vi "Gif.Main.vi"(0 "file path":path, 9 "bgcolor":u32(colorbox)=16777226, 11 "error in (no error)":errorcluster, 12 "image index":i32) -> (4 "fileData":string, 6 "time":u32[](array[numeric]), 8 "images out":picture[](array[picture]), 13 "image data":T1, 14 "image size":cluster{"Width":u32, "Height":u32}, 15 "error out":errorcluster)   [LabVIEW 2019]
doc: "This VI reads all images from a gif file.\nCurrently it can only read from version 89a.\nInterlaced images are not taken into account.\n\nThe outputs are an array of all delay times, an array of all images, the image size and an error cluster.\n\nVersion 01.01\nMike Schröder"
uses:
  <vilib>/picture/picture.llb/imagedata.ctl
panel:
  out "color table":u32[](array[colorbox])
  out "Version":string
  out "Signature":string
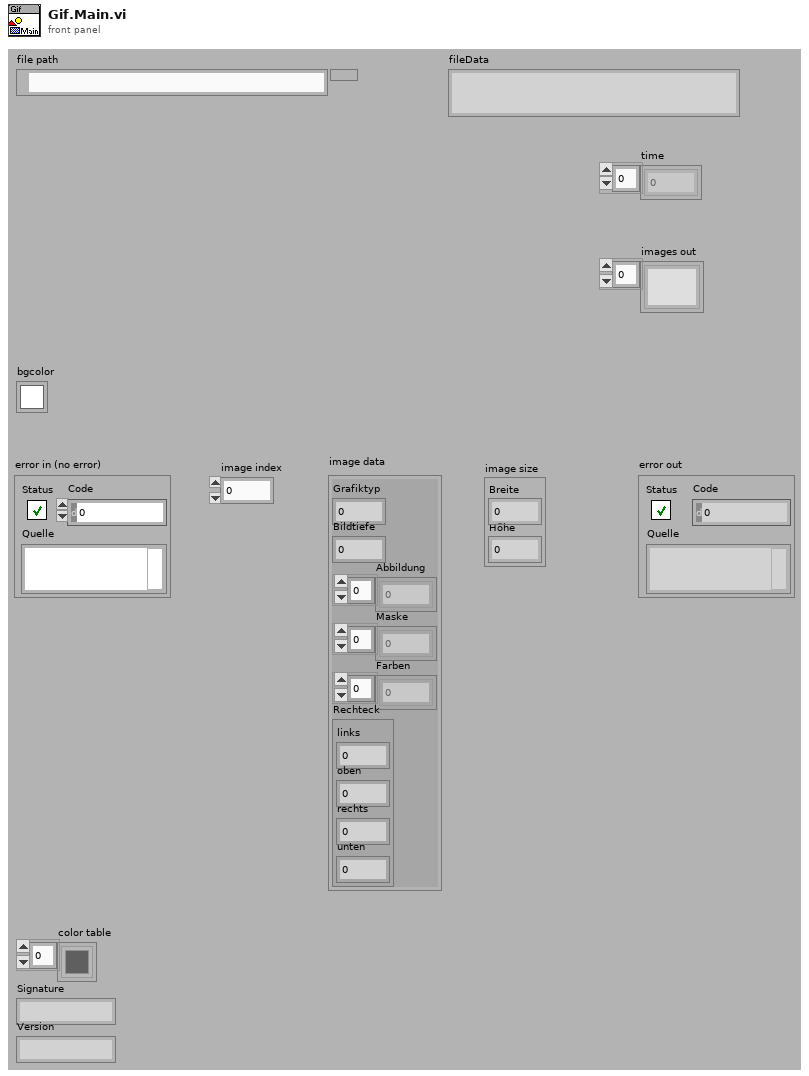
[diagram p1: front panel]
types:
  T1 = typedef "imagedata.ctl" = cluster{"image type":i32, "image depth":i32, "image":u8[], "mask":u8[], "colors":u32[], "Rectangle":cluster{"left":i16, "top":i16, "right":i16, "bottom":i16}}
  T2 = enum16{"deny read/write", "deny write-only", "deny none"}
  T3 = enum16{"read/write", "read-only", "write-only", "write-only (truncate)"}
  T4 = typedef "Gif.LogicalScreenDescriptior.ctl" = cluster{"Logical Screen Width":u16, "Logical Screen Height":u16, "Global Color Table Flag":u8, "Color Resolution":u8, "Sort Flag":u8, "Size of Global Color Table":u8, "Background Color Index":u8, "Pixel Aspect Ratio":u8}
  T5 = typedef "Gif.GraphicControlExtension.ctl" = cluster{"Reserved":u8, "Disposal Method":u8, "User Input Flag":u8, "Transparent Color Flag":u8, "Delay Time":u16, "Transparent Color Index":u8}
  T6 = typedef "Gif.ImageDescriptor.ctl" = cluster{"Image Left Position":u16, "Image Top Position":u16, "Image Width":u16, "Image Height":u16, "Local Color Table Flag":u8, "Interlace Flag":u8, "Sort Flag":u8, "Reserved":u8, "Size Of Local Color Table":u8}
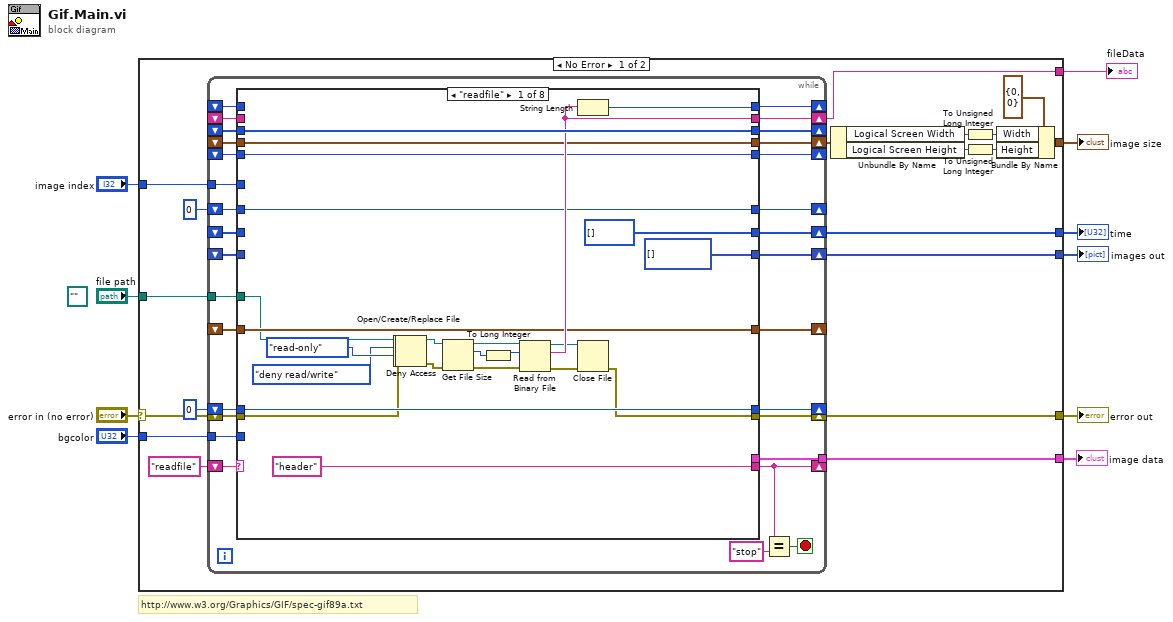
[diagram p0: block diagram]
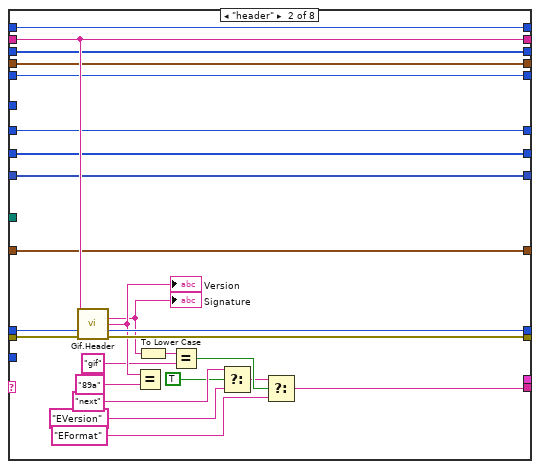
[diagram p2: hidden frame]
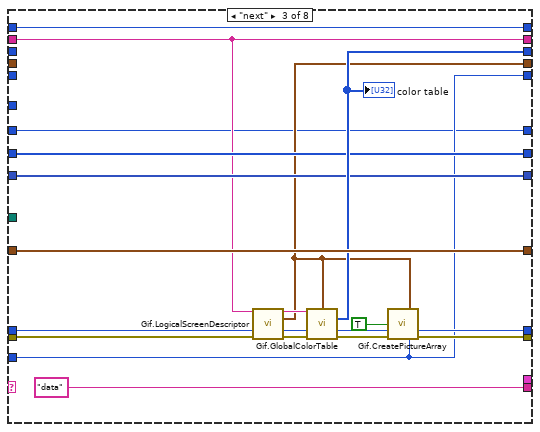
[diagram p3: hidden frame]
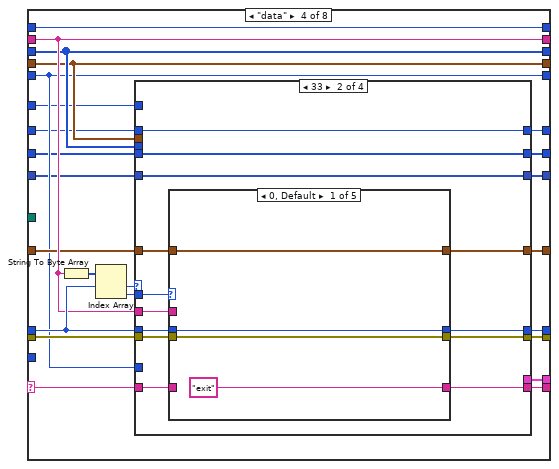
[diagram p4: hidden frame]
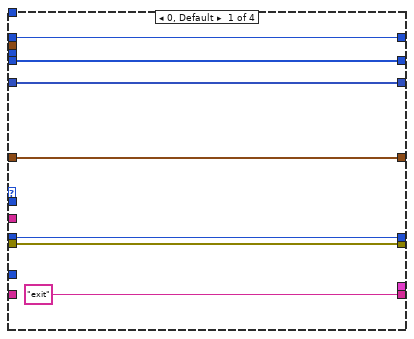
[diagram p5: hidden frame]
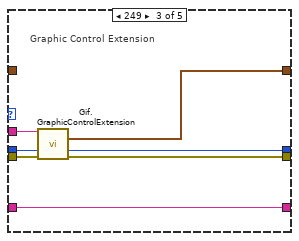
[diagram p7: hidden frame]
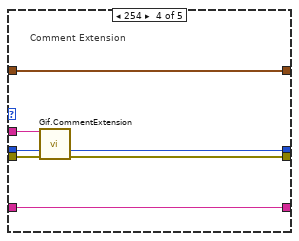
[diagram p8: hidden frame]
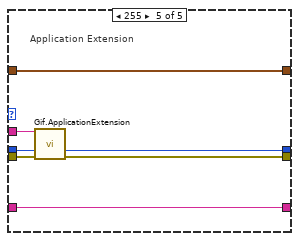
[diagram p9: hidden frame]
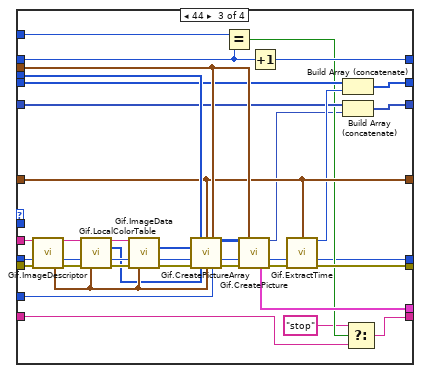
[diagram p10: hidden frame]
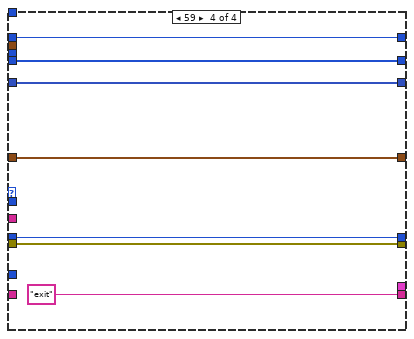
[diagram p11: hidden frame]
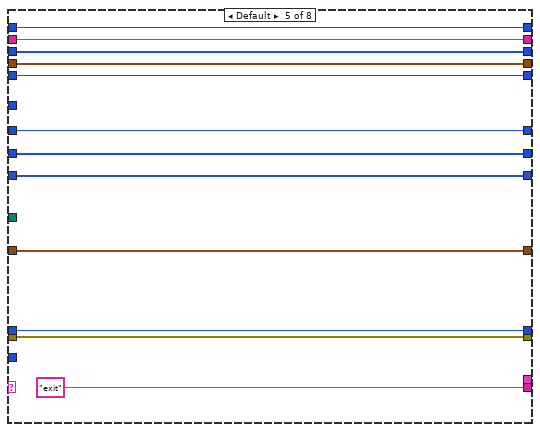
[diagram p12: hidden frame]
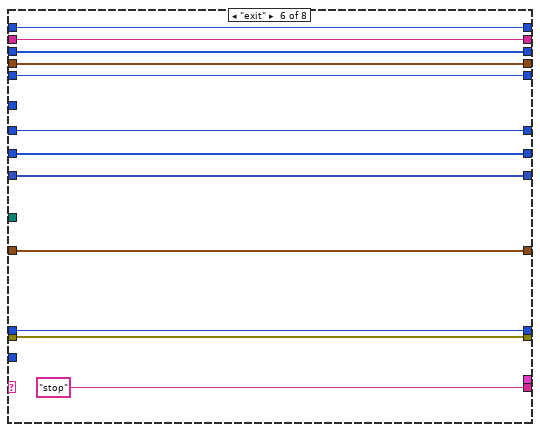
[diagram p13: hidden frame]
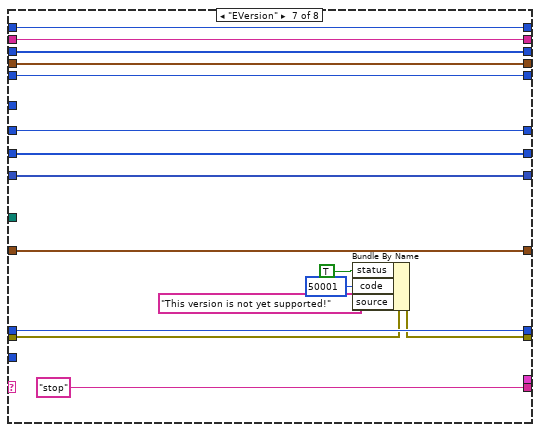
[diagram p14: hidden frame]
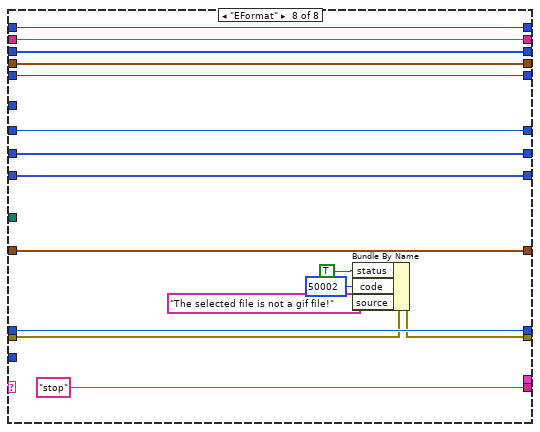
[diagram p15: hidden frame]
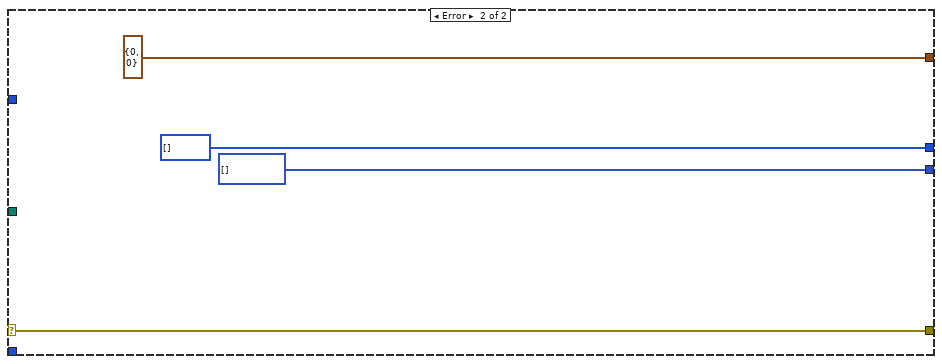
[diagram p16: hidden frame]
diagram:
  (unwired) path "" ("file path")
  # "http://www.w3.org/Graphics/GIF/spec-gif89a.txt"
  n1 = case shown="No Error" "error in (no error)" {
    selector: "error in (no error)" -> [w15 w309]
    tunnel: [w27 u32[] []] -> w10
    tunnel: [w26 picture[] []] -> w2
    tunnel: "bgcolor" -> [w24 _]
    tunnel: "file path" -> [w23 _]
    tunnel: [w22 w309] -> w7
    tunnel: [w16 cluster{"Width":u32, "Height":u32} {"Width"=0, "Height"=0} ("Größe des Darstellungsbereichs")] -> w6
    tunnel: "image index" -> [w13 _]
    tunnel: [w12 _] -> w3
    tunnel: [w11 _] -> w1
    frame No Error {
      n2 = while {
        shift-right: [w50] -> _
        shift-left: "readfile" -> [w59]
        shift-right: [w58] -> _
        shift-left: _ -> [w56]
        shift-right: [w57] -> w11
        shift-left: _ -> [w55]
        shift-right: [w53] -> w22
        shift-left: w15 -> [w54]
        shift-right: [w51] -> _
        shift-left: 0 ("offset (0)") -> [w52]
        shift-right: [w47] -> _
        shift-left: _ -> [w46]
        shift-right: [w45] -> _
        shift-left: _ -> [w44]
        shift-right: [w43] -> w25
        shift-left: _ -> [w42]
        shift-right: [w41] -> _
        shift-left: _ -> [w40]
        shift-right: [w38] -> w27
        shift-left: _ -> [w39]
        shift-right: [w36] -> w26
        shift-left: _ -> [w37]
        tunnel: w24 -> [w35]
        tunnel: w23 -> [w34]
        shift-right: [w31] -> _
        shift-left: 0 ("offset (0)") -> [w32]
        tunnel: w13 -> [w30]
        tunnel: [w33] -> w12
        stop <- w48 stop-if-true
        n3 = case shown="\"readfile\"" w59 {
          selector: w59 -> [_ _ _ w145 _ _ _ _]
          tunnel: [w85 w110 w130 w154 w261 w273 w289 w305] -> w58
          tunnel: [w81 w108 w114 w144 w260 w272 w288 w304] -> w57
          tunnel: w56 -> [_ w110 w130 w154 w261 w273 w289 w305]
          tunnel: w55 -> [_ w108 w114 w144 w260 w272 w288 w304]
          tunnel: ["header" w89 "data" w146 "exit" "stop" "stop" "stop"] -> w50
          tunnel: w54 -> [w73 w109 w113 w149 w258 w270 w279 w295]
          tunnel: [w60 w103 w117 w148 w258 w270 w278 w294] -> w53
          tunnel: w52 -> [w83 w107 w112 w150 w257 w269 w286 w302]
          tunnel: [w83 w102 w119 w147 w257 w269 w286 w302] -> w51
          tunnel: [w82 w101 w124 w143 w256 w268 w285 w301] -> w47
          tunnel: w46 -> [w82 w101 _ w143 w256 w268 w285 w301]
          tunnel: [w78 w106 w128 w142 w255 w267 w284 w300] -> w45
          tunnel: w44 -> [w78 w106 w128 w141 w255 w267 w284 w300]
          tunnel: [w77 w100 w116 w140 w254 w266 w283 w299] -> w43
          tunnel: w42 -> [w77 w100 _ w140 w254 w266 w283 w299]
          tunnel: [w76 w99 w115 w139 w253 w265 w282 w298] -> w41
          tunnel: w40 -> [w76 w99 _ w139 w253 w265 w282 w298]
          tunnel: w39 -> [_ w105 w123 w138 w252 w264 w281 w297]
          tunnel: [u32[] [] w105 w123 w137 w252 w264 w281 w297] -> w38
          tunnel: w37 -> [_ w104 w122 w136 w251 w263 w280 w296]
          tunnel: [picture[] [] w104 w122 w135 w251 w263 w280 w296] -> w36
          tunnel: w35 -> [_ _ w115 _ _ _ _ _]
          tunnel: w34 -> [w74 _ _ _ _ _ _ _]
          tunnel: [_ _ _ w134 _ _ _ _] -> w33
          tunnel: w32 -> [w72 w86 w111 w133 w250 w262 w274 w290]
          tunnel: [w72 w86 w111 w132 w250 w262 w274 w290] -> w31
          tunnel: w30 -> [_ _ _ w131 _ _ _ _]
          frame "readfile" {
            n4 = Open/Create/Replace File(file path (use dialog)=w74, error in=w73, access (0:read/write)=T3."read-only" ("open mode (0)")) -> (refnum out=w63:refnum<file>, error out=w64:errorcluster)  [unwired: 3 in, 1 out]
            n5 = Deny Access(4:w64, 6:T2."deny read/write" ("deny mode (2)"), 7:w63) -> (0:w69:errorcluster, 3:w70:refnum<file>)
            n6 = Get File Size(file=w70, error in=w69) -> (refnum out=w79:refnum<file>, size (in bytes)=w65:i64, 0:w80:errorcluster)
            n7 = To Long Integer(number=w65) -> (32bit integer=w68:i32)
            n8 = Read from Binary File(8:w80, 10:w68, 11:w79) -> (0:w61:errorcluster, 2:w81:string, 3:w62:refnum<file>)  [unwired: 3 in, 1 out]
            n9 = String Length(string=w81) -> (length=w85:i32)
            n10 = Close File(refnum=w62, error in=w61) -> (error out=w60:errorcluster)  [unwired: 1 out]
          }
          frame "header" {
            n11 = call "Gif.Header.vi"("data"=w108, "offset"=w107, "error in (no error)"=w109) -> ("Signature"=w94:string, "Version"=w98:string, "offset out"=w102:i32, "error out"=w103:errorcluster)  [unwired: 1 in, 8 out]
            "Signature" <- w94
            "Version" <- w98
            n12 = Equal?(x=w98, y="89a") -> ()  [unwired: 1 out]
            n13 = To Lower Case(string=w94) -> (all lower case string=w93:string)
            n14 = Equal?(x=w93, y="gif") -> (x = y?=w91:bool)
            n15 = Select(t="next", s=TRUE, f="EVersion") -> (s? t:f=w90:string)
            n16 = Select(t=w90, s=w91, f="EFormat") -> (s? t:f=w89:string)
          }
          frame "next" {
            n17 = call "Gif.LogicalScreenDescriptor.vi"("data"=w114, "offset"=w112, "error in (no error)"=w113) -> ("data out"=w125:string, "Logical Screen Descriptor"=w116:T4, "offset out"=w126:i32, "error out"=w127:errorcluster)  [unwired: 9 out]
            n18 = call "Gif.GlobalColorTable.vi"("data"=w125, "Logical Screen Descriptor"=w116, "offset"=w126, "error in (no error)"=w127) -> ("global color table"=w124:u32[], "offset out"=w120:i32, "error out"=w118:errorcluster)  [unwired: 1 in, 8 out]
            "color table" <- w124
            n19 = call "Gif.CreatePictureArray.vi"("Logical Screen Description"=w116, "init"=TRUE, "offset"=w120, "error in (no error)"=w118, "bgcolor"=w115) -> ("offset out"=w119:i32, "error out"=w117:errorcluster)  [unwired: 5 in, 4 out]
          }
          frame "data" {
            n20 = String To Byte Array(string=w144) -> (unsigned byte array=w153:u8[])
            n21 = Index Array(array=w153, index #1=w150) -> (element #1=w152:u8, element #2=w151:u8)  [unwired: 1 in]
            n22 = case shown="33" w152 {
              tunnel: w151 -> [_ w174 _ _]
              tunnel: w150 -> [w160 w170 w241 w248]
              tunnel: w149 -> [w161 w169 w242 w247]
              tunnel: [w161 w168 w216 w247] -> w148
              tunnel: [w160 w171 w206 w248] -> w147
              tunnel: ["exit" w173 w208 "exit"] -> w146
              tunnel: w145 -> [_ w172 w210 _]
              tunnel: w144 -> [_ w167 w240 _]
              tunnel: w143 -> [_ _ w226 _]
              tunnel: [w158 w166 w224 w246] -> w142
              tunnel: w141 -> [w158 w165 w224 w246]
              tunnel: w140 -> [_ _ w225 _]
              tunnel: w139 -> [_ _ w223 _]
              tunnel: w138 -> [w157 w164 w222 w245]
              tunnel: [w157 w164 w220 w245] -> w137
              tunnel: w136 -> [w156 w163 w219 w244]
              tunnel: [w156 w163 w218 w244] -> w135
              tunnel: [_ _ w214 _] -> w134
              tunnel: w133 -> [w155 w162 w204 w243]
              tunnel: [w155 w162 w212 w243] -> w132
              tunnel: w131 -> [_ _ w213 _]
              frame 0, Default {
              }
              frame 33 {
                n23 = case shown="0, Default" w174 {
                  tunnel: ["exit" w182 w189 w196 w203] -> w173
                  tunnel: w172 -> [_ w182 w189 w196 w203]
                  tunnel: [w177 w181 w185 w193 w201] -> w171
                  tunnel: w170 -> [w177 w181 w187 w194 w202]
                  tunnel: w169 -> [w176 w180 w188 w195 w200]
                  tunnel: [w176 w180 w186 w192 w199] -> w168
                  tunnel: w167 -> [_ _ w184 w191 w198]
                  tunnel: [w175 w179 w183 w190 w197] -> w166
                  tunnel: w165 -> [w175 w179 _ w190 w197]
                  frame 0, Default {
                  }
                  frame 1 {
                  }
                  frame 249 {
                    # "Graphic Control Extension"
                    n24 = call "Gif.GraphicControlExtension.vi"("data"=w184, "offset"=w187, "error in (no error)"=w188) -> ("GraphicControlExtension"=w183:T5, "offset out"=w185:i32, "error out"=w186:errorcluster)  [unwired: 10 out]
                  }
                  frame 254 {
                    # "Comment Extension"
                    n25 = call "Gif.CommentExtension.vi"("data"=w191, "offset"=w194, "error in (no error)"=w195) -> ("offset out"=w193:i32, "error out"=w192:errorcluster)  [unwired: 11 out]
                  }
                  frame 255 {
                    # "Application Extension"
                    n26 = call "Gif.ApplicationExtension.vi"("data"=w198, "offset"=w202, "error in (no error)"=w200) -> ("offset out"=w201:i32, "error out"=w199:errorcluster)  [unwired: 11 out]
                  }
                }
              }
              frame 44 {
                n27 = call "Gif.ImageDescriptor.vi"("data"=w240, "offset"=w241, "error in (no error)"=w242) -> ("data out"=w237:string, "offset out"=w238:i32, "ImageDescriptor"=w228:T6, "error out"=w239:errorcluster)  [unwired: 9 out]
                n28 = call "Gif.LocalColorTable.vi"("data"=w237, "offset"=w238, "error in (no error)"=w239, "ImageDescriptor"=w228) -> ("data out"=w234:string, "local color table"=w227:u32[], "offset out"=w235:i32, "error out"=w236:errorcluster)  [unwired: 5 in, 3 out]
                n29 = call "Gif.ImageData.vi"("data"=w234, "offset"=w235, "error in (no error)"=w236, "ImageDescriptor"=w228) -> ("Index Array"=w232:i32[], "offset out"=w207:i32, "error out"=w233:errorcluster)  [unwired: 1 in, 8 out]
                n30 = call "Gif.CreatePictureArray.vi"("gloal color table"=w226, "GraphicControlExtension"=w224, "Logical Screen Description"=w225, "Index Array"=w232, "offset"=w207, "error in (no error)"=w233, "local color table"=w227, "ImageDescriptor"=w228, "bgcolor"=w223) -> ("image out"=w229:u32[][], "offset out"=w230:i32, "error out"=w231:errorcluster)  [unwired: 1 in, 3 out]
                n31 = Equal?(x=w213, y=w204) -> (x = y?=w211:bool)
                n32 = call "Gif.CreatePicture.vi"("image in"=w229, "Logical Screen Description"=w225, "offset"=w230, "error in (no error)"=w231) -> ("image out"=w205:picture, "offset out"=w215:i32, "graphic data"=w214:T1, "error out"=w217:errorcluster)  [unwired: 8 out]
                n33 = Increment(x=w204) -> (x+1=w212:i32)
                n34 = call "Gif.ExtractTime.vi"("GraphicControlExtension"=w224, "offset"=w215, "error in (no error)"=w217) -> ("time"=w221:u32, "offset out"=w206:i32, "error out"=w216:errorcluster)  [unwired: 10 out]
                n35 = Build Array (concatenate)(w222, w221) -> (w220:u32[])
                n36 = Build Array (concatenate)(w219, w205) -> (w218:picture[])
                n37 = Select(t="stop", s=w211, f=w210) -> (s? t:f=w208:string)
              }
              frame 59 {
              }
            }
          }
          frame Default {
          }
          frame "exit" {
          }
          frame "EVersion" {
            n38 = Bundle By Name(cluster=w279, "status"=TRUE, "code"=50001, "source"="This version is not yet supported!") -> (w278:errorcluster)
          }
          frame "EFormat" {
            n39 = Bundle By Name(cluster=w295, "status"=TRUE, "code"=50002, "source"="The selected file is not a gif file!") -> (w294:errorcluster)
          }
        }
        n40 = Equal?(x=w50, y="stop") -> (x = y?=w48:bool)
      }
      n41 = Unbundle By Name(w25) -> ("Logical Screen Width"=w19:u16, "Logical Screen Height"=w18:u16)
      n42 = To Unsigned Long Integer(number=w19) -> (unsigned 32bit integer=w20:u32)
      n43 = To Unsigned Long Integer(number=w18) -> (unsigned 32bit integer=w21:u32)
      n44 = Bundle By Name(cluster=cluster{"Width":u32, "Height":u32} {"Width"=0, "Height"=0} ("Größe des Darstellungsbereichs"), "Width"=w20, "Height"=w21) -> (w16:cluster{"Width":u32, "Height":u32})
    }
    frame Error {
    }
  }
  "time" <- w10
  "error out" <- w7
  "image size" <- w6
  "image data" <- w3
  "images out" <- w2
  "fileData" <- w1
